vi "led control loop.vi"() -> (0 "error out":errorcluster, 2 "Command":string, 3 "I2C Byte Output Array":u8[](array[numeric]))   [LabVIEW 2014]
uses:
  <vilib>/Rock Robotics/WPI/DriverStation/WPI_DriverStationAllianceInfo.ctl
  <vilib>/Rock Robotics/WPI/DriverStation/WPI_DriverStationRobotMode2.ctl
  global variables/devrefs.vi
panel:
  # "LED Control for the Robot's LEDs Through an Arduino"
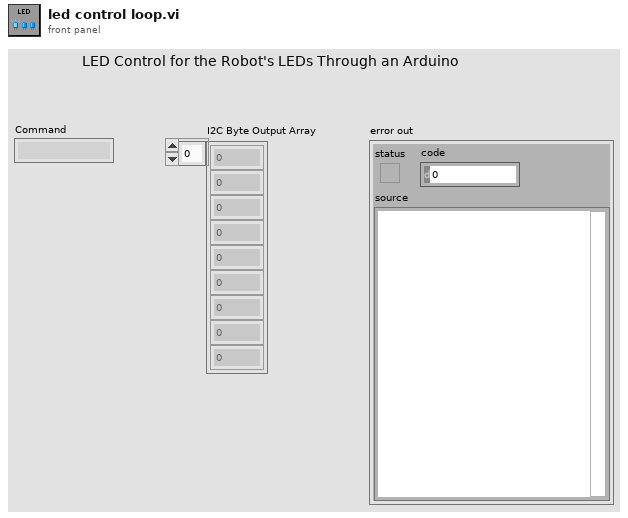
[diagram p1: front panel]
types:
  T1 = typedef "WPI_DriverStationRobotMode2.ctl" = enum16{"Autonomous Disabled", "Autonomous Enabled", "Teleop Disabled", "Teleop Enabled", "Disconnected", "Finish", "Test Disabled", "Test Enabled", "Emergency Stopped"}
  T2 = typedef "WPI_DriverStationAllianceInfo.ctl" = enum16{"Red", "Blue", "Invalid"}
  T3 = typedef "WPI_EncoderDevRef.ctl" = cluster{"DevStatus":errorcluster, "EncoderIndex":T4, "CounterIndex":T5, "DistancePerCount":dbl, "Decoding Type":T6}
  T4 = typedef "FPGA_EncoderIdx.ctl" = enum8{"Enc 0", "Enc 1", "Enc 2", "Enc 3", "Enc 4", "Enc 5", "Enc 6", "Enc 7", "Invalid"}
  T5 = typedef "FPGA_CounterCtrSystemIndex.ctl" = enum8{"Ctr 0", "Ctr 1", "Ctr 2", "Ctr 3", "Ctr 4", "Ctr 5", "Ctr 6", "Ctr 7", "Invalid"}
  T6 = typedef "WPI_EncoderType.ctl" = enum16{"1x", "2x", "4x"}
  T7 = typedef "WPI_I2CDevRef.ctl" = cluster{"DevStatus":errorcluster, "Controller":T8, "Device Address":u8, "Handle":i32, "I2C Bus":T9}
  T8 = typedef "FPGA_TypedefDigitalModule.ctl" = enum16{"Controller 1"}
  T9 = typedef "i2c_bus.ctl" = enum16{"I2C On-Board", "I2C MXP", "Invalid"}
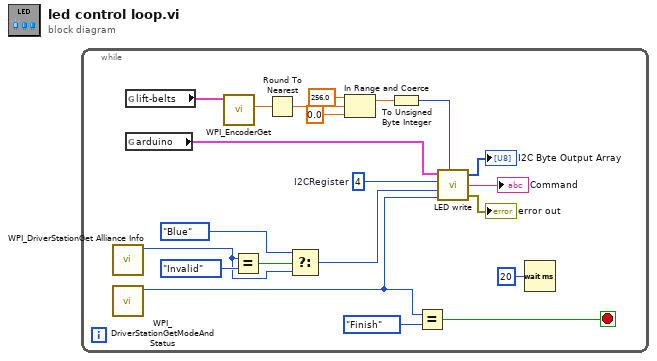
[diagram p0: block diagram]
diagram:
  n1 = while {
    stop <- w4 stop-if-true
    w8 = u8 4  # I2CRegister
    n2 = call <vilib>:"WPI_DriverStationGet Alliance Info.vi"() -> ("Alliance"=w12:T2)  [unwired: 10 in, 1 out]
    n3 = call <vilib>:"WPI_DriverStationGetModeAndStatus.vi"() -> ("Robot Mode"=w6:T1)  [unwired: 10 in, 1 out]
    n4 = global read "devrefs.vi" "lift-belts"() -> (w21:T3)
    n5 = global read "devrefs.vi" "arduino"() -> (w9:T7)
    n6 = call <vilib>:"WPI_EncoderGet.vi"("EncoderDevRef"=w21) -> ("Distance"=w20:dbl)  [unwired: 5 in, 5 out]
    n7 = Equal?(x=w12, y=WPI_DriverStationAllianceInfo."Invalid") -> (x = y?=w13:bool)
    n8 = Round To Nearest(number=w20) -> (nearest integer value=w19:dbl)
    n9 = Select(t=WPI_DriverStationAllianceInfo."Blue", s=w13, f=w12) -> (s? t:f=w10:T2)
    n10 = In Range and Coerce(upper limit=256.0, x=w19, lower limit=0.0) -> (coerced(x)=w16:dbl)  [unwired: 1 out]
    n11 = To Unsigned Byte Integer(number=w16) -> (unsigned 8bit integer=w15:u8)
    n12 = Equal?(x=w6, y=WPI_DriverStationRobotMode2."Finish") -> (x = y?=w4:bool)
    n13 = call "LED write.vi"("I2CDevRef"=w9, "I2CRegister"=w8, "Alliance"=w10, "Robot Mode"=w6, "Lift Position"=w15) -> ("I2C Byte Output Array"=→"I2C Byte Output Array":u8[], "Command"=→"Command":string, "error out"=→"error out":errorcluster)
    n14 = Wait (ms)(milliseconds to wait=u32 20) -> ()  [unwired: 1 out]
  }
